vi "IV6.3MV4.PMDD.vi"() -> ()   [LabVIEW 2019]
uses:
  IV6.3MV4.PMDD_NAVEGACION.vi
panel:
  in  "NIP_INSTRUCCIONES_str":string[](array[string])
  out "appended array":string[](array[string])
  out "appended array 2":string[](array[string])
  out "String":string
  out "3 segundos":i32
  out "x-y*floor(x/y)":i32
  out "while i":i32
  in  "Insertar Tarjeta":bool
  out "NAVEGACION":T1
  out "LED":bool
  out "TABS_IMGs":enum32{"IMG1", "IMG2", "IMG3"}(tab) caption="Tab Control 2"
  in  "NIP":string
  in  "ACEPTAR":bool
  out "NIP INTRUCCIONES ARRAY indicator":string
  in  "Stop Button":bool
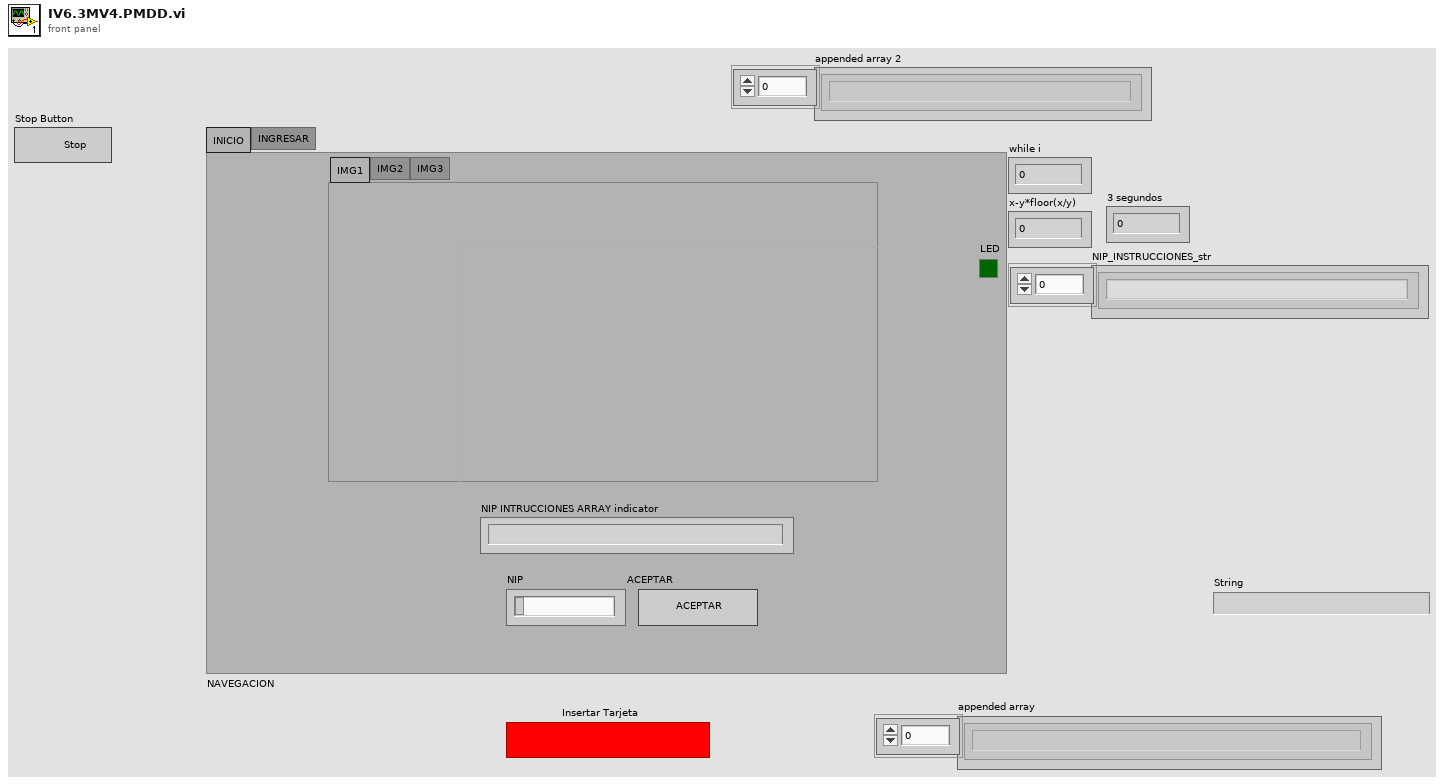
[diagram p1: front panel]
types:
  T1 = typedef "IV6.3MV4.PMDD_NAVEGACION.vi" = enum32{"INICIO", "INGRESAR"}
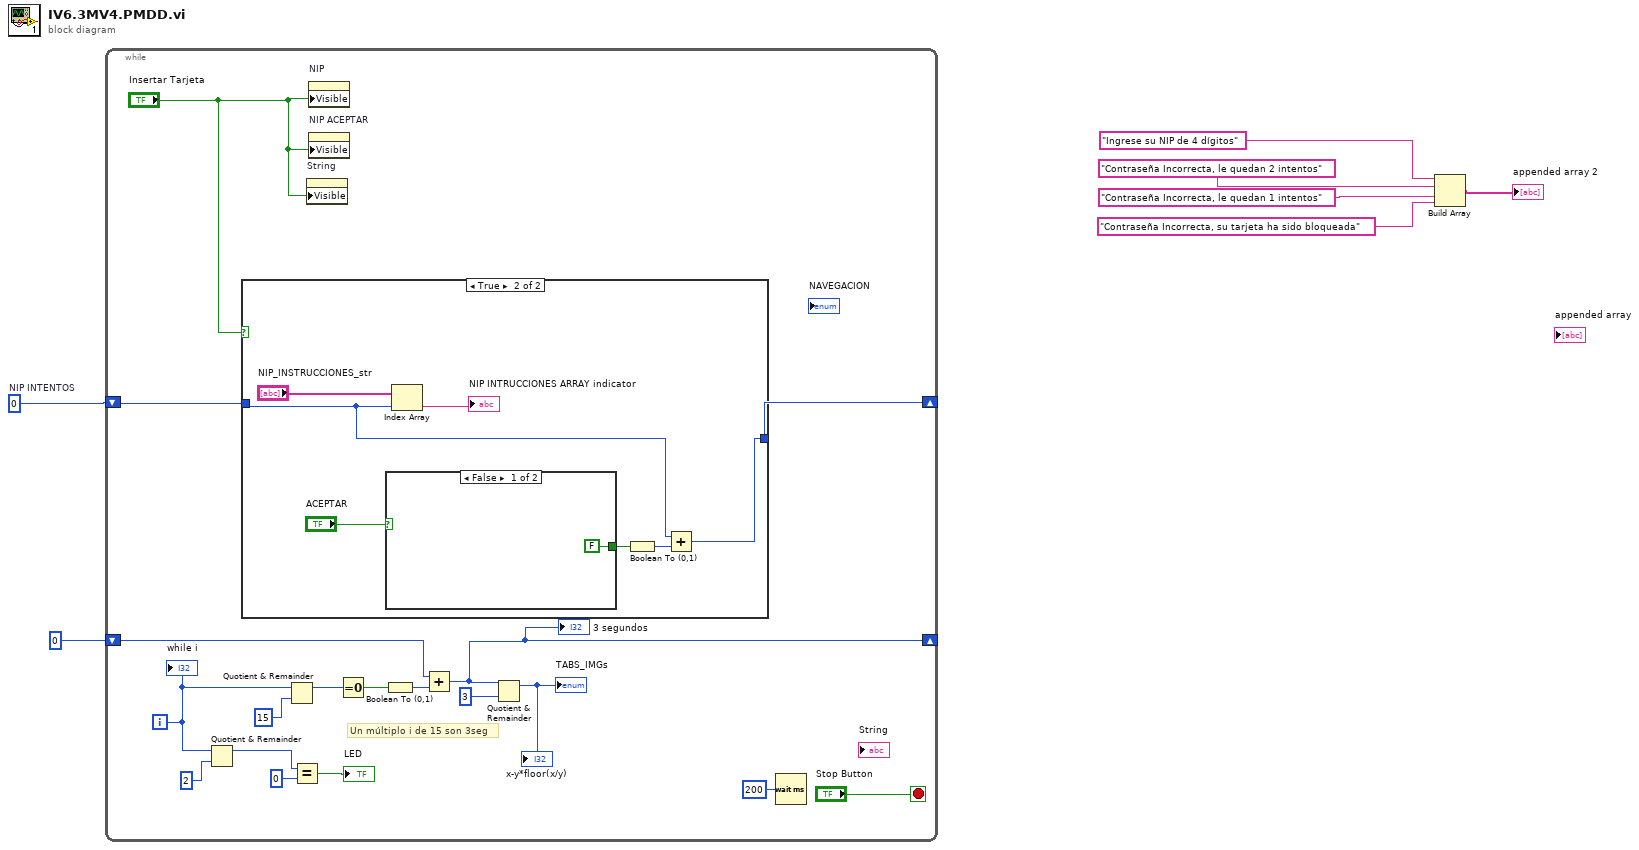
[diagram p0: block diagram]
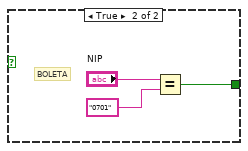
[diagram p3: hidden frame]
diagram:
  w1 = 0  # NIP INTENTOS
  n1 = while {
    shift-right: [w12] -> _
    shift-left: 0 -> [w13]
    shift-right: [w8] -> _
    shift-left: w1 -> [w9]
    i -> [w17]
    stop <- "Stop Button" stop-if-true
    # "Un múltiplo i de 15 son 3seg"
    n2 = Quotient & Remainder(x=w17, y=2) -> (x-y*floor(x/y)=w20:i32)  [unwired: 1 out]
    n3 = case shown="True" "Insertar Tarjeta" {
      tunnel: w9 -> [w26 w28]
      tunnel: [w26 w27] -> w8
      frame False {
      }
      frame True {
        n4 = case shown="False" "ACEPTAR" {
          tunnel: [FALSE w35] -> w30
          frame False {
          }
          frame True {
            # "BOLETA"
            n5 = Equal?(x="NIP", y="0701") -> (x = y?=w35:bool)
          }
        }
        n6 = Index Array(array="NIP_INSTRUCCIONES_str", index=w28) -> (element=→"NIP INTRUCCIONES ARRAY indicator":string)
        n7 = Boolean To (0,1)(Boolean=w30) -> (0, 1=w29:i16)
        n8 = Add(x=w28, y=w29) -> (x+y=w27:i32)
      }
    }
    n9 = Quotient & Remainder(x=w17, y=15) -> (x-y*floor(x/y)=w16:i32)  [unwired: 1 out]
    n10 = Equal?(x=w20, y=0) -> (x = y?=→"LED":bool)
    n11 = property on="String" class="Str"("Visible"="Insertar Tarjeta") -> ()  [unwired: 2 in, 2 out]
    n12 = property on="NIP" class="Str"("Visible"="Insertar Tarjeta") -> ()  [unwired: 2 in, 2 out]
    n13 = property on="NIP ACEPTAR" class="Bool (strict)"("Visible"="Insertar Tarjeta") -> ()  [unwired: 2 in, 2 out]
    n14 = Equal To 0?(x=w16) -> (x = 0?=w15:bool)
    n15 = Boolean To (0,1)(Boolean=w15) -> (0, 1=w14:i16)
    n16 = Add(x=w13, y=w14) -> (x+y=w12:i32)
    "3 segundos" <- w12
    n17 = Quotient & Remainder(x=w12, y=3) -> (x-y*floor(x/y)=→"TABS_IMGs" →"x-y*floor(x/y)":i32)  [unwired: 1 out]
    n18 = Wait (ms)(milliseconds to wait=u32 200) -> ()  [unwired: 1 out]
    "while i" <- w17
  }
  n19 = Build Array("Ingrese su NIP de 4 dígitos", "Contraseña Incorrecta, le quedan 2 intentos", "Contraseña Incorrecta, le quedan 1 intentos", "Contraseña Incorrecta, su tarjeta ha sido bloqueada") -> (→"appended array 2":string[])
